vi "配置文件读写.vi"(8 "error in (no error)":errorcluster caption="错误输入（无错误）", 10 "write?":bool, 11 "HTTP发送 输入":refnum<class "HTTP发送.lvclass">) -> (0 "error out":errorcluster caption="错误输出", 3 "HTTP发送 输出":refnum<class "HTTP发送.lvclass">)   [LabVIEW 2022 SP3, in "工况数据上传.lvlib" / "HTTP发送.lvclass"]
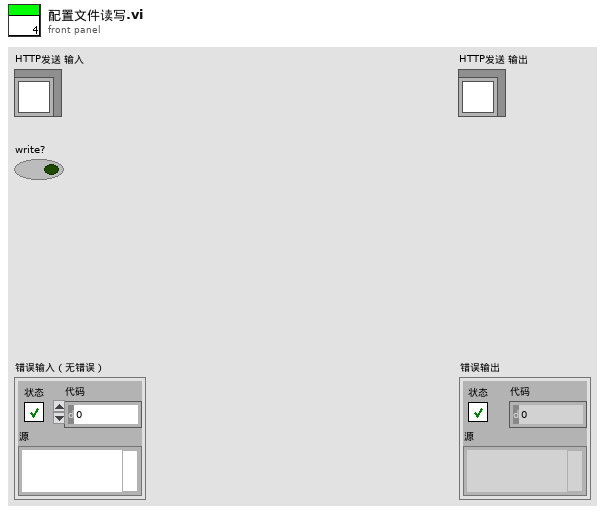
[diagram p1: front panel]
types:
  T1 = cluster{"url":string, "loginTokenRequest":cluster{"clientId":string, "clientSecret":string, "grantType":string, "password":string, "scope":string, "userName":string, "userType":string}, "自动获取MN":bool}
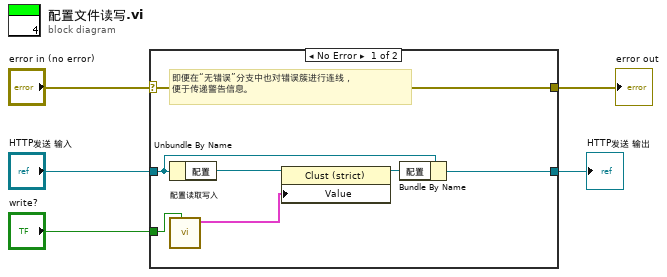
[diagram p0: block diagram]
diagram:
  n1 = case shown="No Error" "error in (no error)" {
    selector: "error in (no error)" -> [w12 w14]
    tunnel: [w12 w14] -> w4
    tunnel: [w6 w13] -> w2
    tunnel: "HTTP发送 输入" -> [w8 w13]
    tunnel: "write?" -> [w9 _]
    frame No Error {
      # "即便在“无错误”分支中也对错误簇进行连线，\n便于传递警告信息。"
      n2 = Unbundle By Name(w8) -> ("配置"=w11:refnum<vi>)
      n3 = call "配置读取写入.vi"("write"=w9) -> ("配置输出"=w10:T1)  [unwired: 9 in, 1 out]
      n4 = property class="Clust (strict)"(reference=w11, "Value"=w10) -> (reference out=w7:refnum<vi>)  [unwired: 1 in, 1 out]
      n5 = Bundle By Name(cluster=w8, "配置"=w7) -> (w6:refnum<class "HTTP发送.lvclass">)
    }
    frame Error {
    }
  }
  "error out" <- w4
  "HTTP发送 输出" <- w2
